vi "Run Refill.vi"(8 "error in (no error)":errorcluster, 9 "auto_switch_valve":bool=TRUE, 10 "flow_rate_uL_s":dbl=200.0, 11 "PHD Ultra in":refnum<class "cetoni.lvclass">) -> (0 "error out":errorcluster, 3 "PHD Ultra out":refnum<class "cetoni.lvclass">)   [LabVIEW 2018, in "cetoni.lvlib" / "cetoni.lvclass"]
uses:
  cetoni.lvclass
  cetoni.lvclass/cetoni.ctl
  Resources/GLOBAL/GLOBAL Time-critical.vi
  <userlib>/QmixLib/QmixLib.lvlib
  Program Files/cetoni/QmixSDK/lib/labview/labbCAN_Pump_API/labbCAN_Pump_API.lvlib
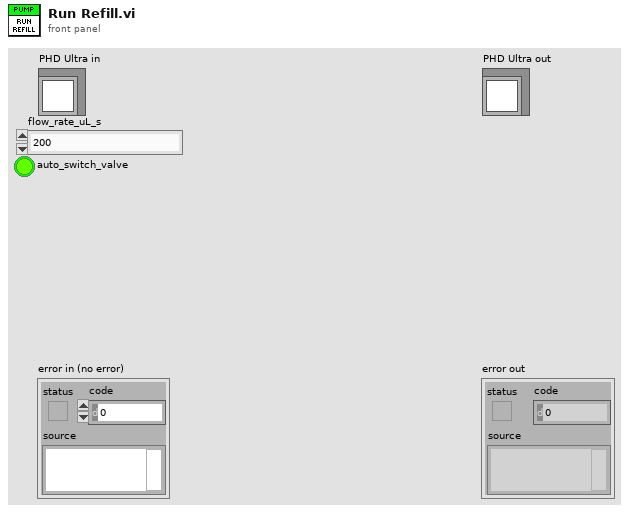
[diagram p1: front panel]
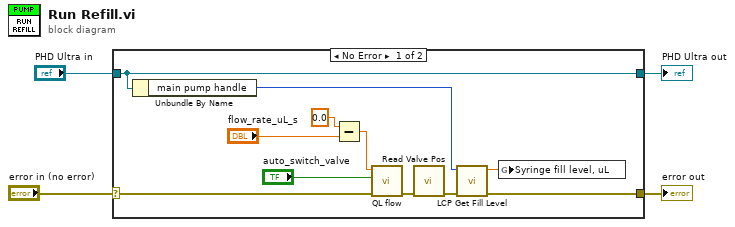
[diagram p0: block diagram]
diagram:
  n1 = case shown="No Error" "error in (no error)" {
    selector: "error in (no error)" -> [w15 w17]
    tunnel: [w5 w17] -> w3
    tunnel: [w8 w16] -> w1
    tunnel: "PHD Ultra in" -> [w8 w16]
    frame No Error {
      n2 = Unbundle By Name(w8) -> ("main pump handle"=w7:i64)
      n3 = Subtract(x=0.0, y="flow_rate_uL_s") -> (x-y=w13:dbl)
      n4 = call <userlib>:"QL flow.vi"("error in (no error)"=w15, "auto_switch_valve"="auto_switch_valve", "flow_rate_uL_s"=w13) -> ("error out"=w10:errorcluster)  [unwired: 8 in]
      n5 = call "Read Valve Pos.vi"("error in (no error)"=w10) -> ("error out"=w6:errorcluster)  [unwired: 10 in]
      n6 = call "LCP Get Fill Level.vi"("error in (no error)"=w6, "Pump Handle"=w7) -> ("error out"=w5:errorcluster, "Fill Level"=w9:dbl)  [unwired: 8 in]
      n7 = global write "GLOBAL Time-critical.vi" "Syringe fill level, uL"(w9) -> ()
    }
    frame Error {
    }
  }
  "error out" <- w3
  "PHD Ultra out" <- w1
